vi "config_DAQmx Task.vi"(7 "Sample Rate":dbl=10000.0 caption="Sample Rate (Hz)" format="%0.2f", 9 "Physical Channel":tag="Dev1/ai0") -> (0 "error out":errorcluster, 1 "timeout":dbl, 2 "taille de bloc d'acquisition":i32, 3 "task out":refnum<k21>)   [LabVIEW 2010]
doc: "Creation et lancement d'une tâche DAQmx d'acquisition analogique.\nLe nombre de pts par bloc est calculé de manière à ce qu'un bloc représente 100ms de signal."
uses:
  <vilib>/DAQmx/create/channels.llb/DAQmx Create Channel (AI-Voltage-Basic).vi
  <vilib>/DAQmx/configure/timing.llb/DAQmx Timing (Sample Clock).vi
panel:
  in  "Maximum Value":dbl=10.0 format="%0.2f"
  in  "Minimum Value":dbl=-10.0 format="%0.2f"
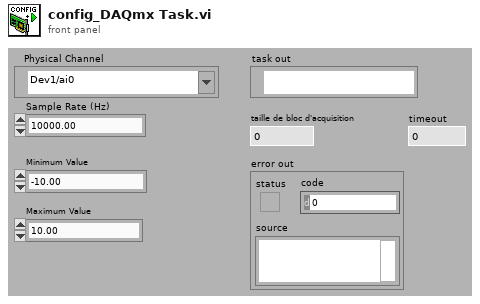
[diagram p1: front panel]
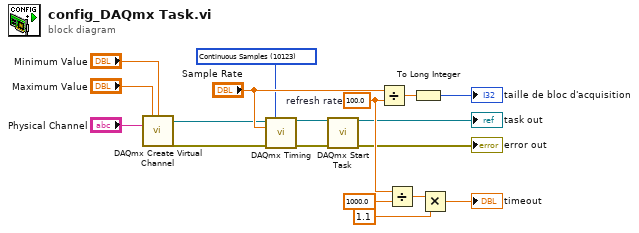
[diagram p0: block diagram]
diagram:
  w14 = 100.0  # refresh rate
  w8 = 10123 items=["Finite Samples"=10178, "Continuous Samples"=10123] ("sample mode")
  n1 = call-poly <vilib>:"DAQmx Create Virtual Channel.vi"("maximum value"="Maximum Value", "minimum value"="Minimum Value", "physical channels"="Physical Channel") -> ("task out"=w5:refnum<k21>, "error out"=w3:errorcluster)  [unwired: 11 in]
  n2 = call-poly <vilib>:"DAQmx Timing.vi"("task/channels in"=w5, "sample mode"=w8, "rate"="Sample Rate", "error in"=w3) -> ("task out"=w9:refnum<k21>, "error out"=w10:errorcluster)  [unwired: 10 in]
  n3 = call <vilib>:"DAQmx Start Task.vi"("task/channels in"=w9, "error in"=w10) -> ("task out"=→"task out":refnum<k21>, "error out"=→"error out":errorcluster)  [unwired: 12 in]
  n4 = Divide(x="Sample Rate", y=w14) -> (x/y=w12:dbl)
  n5 = Divide(x=w14, y=1000.0) -> (x/y=w15:dbl)
  n6 = To Long Integer(number=w12) -> (32bit integer=→"taille de bloc d'acquisition":i32)
  n7 = Multiply(x=w15, y=1.1) -> (x*y=→"timeout":dbl)
